vi "f_gen_with_filter.vi"() -> ()   [LabVIEW 2017]
doc: "This is a signal generator and signal filter combo. It generates a sine wave or a square and includes a high pass filter and a low pass filter. In addition, it can generate mnoise in the signal."
uses:
  typedefs/periodic signal control.ctl
  <vilib>/ptbypt/NI_PtbyPt.lvlib
panel:
  in  "?":enum32{"Signal", "Filter"}(tab)
  in  "Source":T1={"source"=TRUE, "source type"=FALSE, "Amplitude"=1.0, "Period (steps)"=30.0} {"Amplitude" scale=0.0..1.0; "Period (steps)" scale=1.0..1000.0}
  in  "white noise amplitude":dbl(slide)=0.2 scale=0.0..1.0
  in  "white noise":bool
  in  "LP Corner Period":dbl(slide)=50.0 caption="Low Pass Corner Period (steps)" scale=1.0..1000.0
  in  "Low pass":bool=TRUE
  in  "High pass":bool
  in  "HP Corner Period":dbl(slide)=30.0 caption="High Pass Corner Period (steps)" scale=1.0..1000.0
  in  "update interval (ms)":u32(slide)=20 scale=1.0..1000.0
  in  "stop":bool
  out "Waveform Chart":cluster{dbl, dbl}(graph)
  # "Signal Generation and Filtering"
  # "Charles Kinzel\nProject 1\nPhys 350"
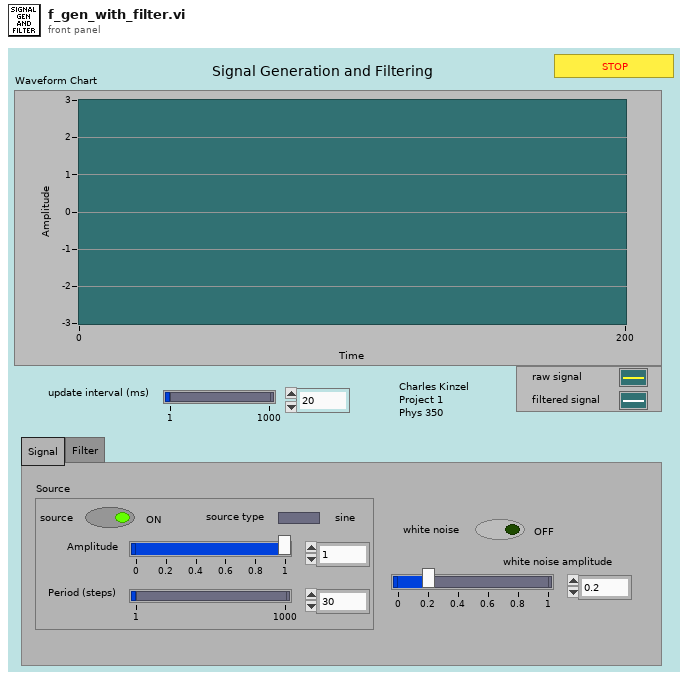
[diagram p1: front panel]
types:
  T1 = typedef "periodic signal control.ctl" = cluster{"source":bool, "source type":bool, "Amplitude":dbl, "Period (steps)":dbl}
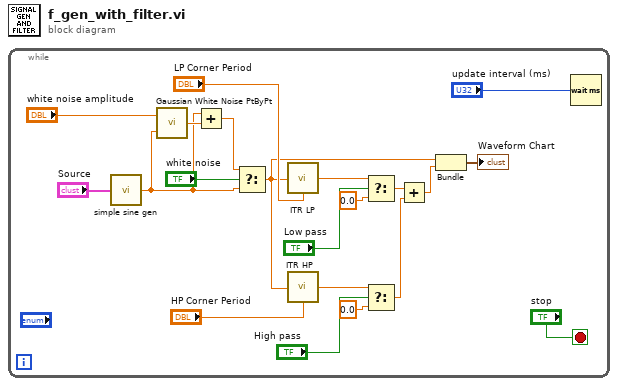
[diagram p0: block diagram]
diagram:
  n1 = while {
    stop <- "stop" stop-if-true
    n2 = call "simple sine gen.vi"("Source"="Source") -> ("output"=w2:dbl)  [unwired: 14 in]
    n3 = call <vilib>:"Gaussian White Noise PtByPt.vi"("seed"=w2, "standard deviation"="white noise amplitude") -> ("Gaussian white noise"=w10:dbl)  [unwired: 1 in]
    n4 = Add(x=w2, y=w10) -> (x+y=w3:dbl)
    n5 = Select(t=w3, s="white noise", f=w2) -> (s? t:f=w1:dbl)
    n6 = call "ITR LP.vi"("input"=w1, "corner period (steps)"="LP Corner Period") -> ("output"=w13:dbl)  [unwired: 13 in]
    n7 = call "ITR HP.vi"("input"=w1, "corner period (steps)"="HP Corner Period") -> ("output"=w12:dbl)  [unwired: 13 in]
    n8 = Select(t=w13, s="Low pass", f=0.0) -> (s? t:f=w9:dbl)
    n9 = Select(t=w12, s="High pass", f=0.0) -> (s? t:f=w8:dbl)
    n10 = Add(x=w9, y=w8) -> (x+y=w7:dbl)
    n11 = Bundle("output"=w1, w7) -> (→"Waveform Chart":cluster{"output":dbl, dbl})  [unwired: 1 in]
    n12 = Wait (ms)(milliseconds to wait="update interval (ms)") -> ()  [unwired: 1 out]
  }
